vi "to_value.vi"(8 "error in (no error)":errorcluster, 11 "Item in":refnum<class "Item.lvclass">) -> (0 "error out":errorcluster, 3 "Value out":refnum<class "Value.lvclass">)   [LabVIEW 2020, in "toml_edit.lvlib" / "Item.lvclass"]
uses:
  Item.lvclass
  Value/Value.lvclass
  Item.lvclass/Item.ctl
  type--enum.ctl
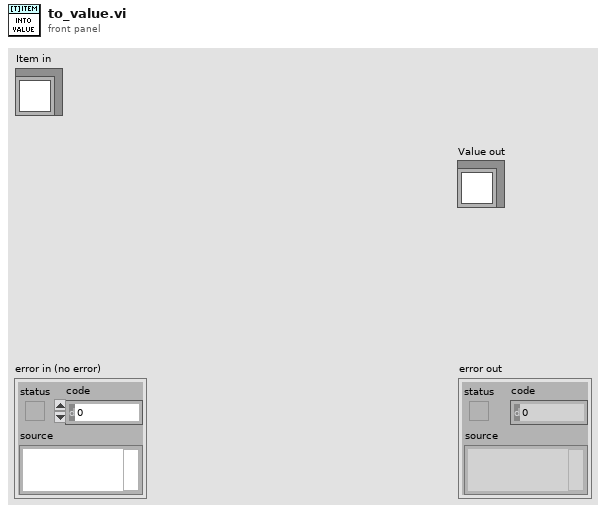
[diagram p1: front panel]
types:
  T1 = typedef "toml_edit.lvlib/Item.lvclass/type--enum.ctl" = enum16{"Unknown", "None", "Value", "ArrayOfTables", "Table"}
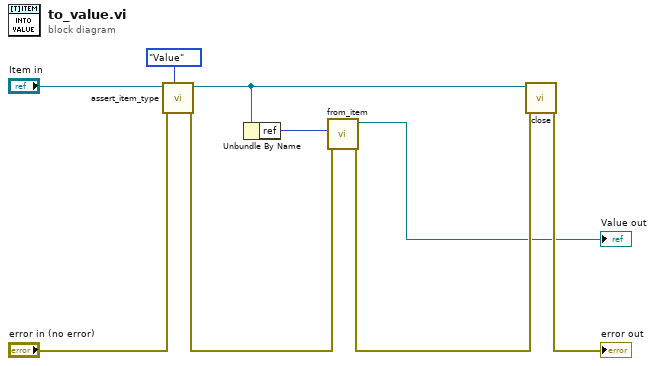
[diagram p0: block diagram]
diagram:
  n1 = call "assert_item_type.vi"("item_type"=type--enum."Value", "error in (no error)"="error in (no error)", "Item in"="Item in") -> ("error out"=w1:errorcluster, "Item out"=w3:refnum<class "Item.lvclass">)  [unwired: 7 in]
  n2 = Unbundle By Name(w3) -> ("ref"=w9:u64)
  n3 = call "from_item.vi"("error in (no error)"=w1, "item_ref"=w9) -> ("error out"=w8:errorcluster, "Value out"=→"Value out":refnum<class "Value.lvclass">)  [unwired: 8 in]
  n4 = call "close.vi"("error in (no error)"=w8, "Item in"=w3) -> ("error out"=→"error out":errorcluster)  [unwired: 9 in]
